vi "AllThingsBaxter_ROS.vi"() -> ()   [LabVIEW 2012]
uses:
  <userlib>/ROSforLV/ROS/MessageBuilding/std_msgs/subs/boolScalar.vi
  <userlib>/ROSforLV/ROS/MessageBuilding/std_msgs/subs/durationScalar.vi
  <userlib>/ROSforLV/ROS/MessageBuilding/std_msgs/subs/float32Scalar.vi
  <userlib>/ROSforLV/ROS/MessageBuilding/std_msgs/subs/float64Scalar.vi
  <userlib>/ROSforLV/ROS/MessageBuilding/std_msgs/subs/i8Scalar.vi
  <userlib>/ROSforLV/ROS/MessageBuilding/std_msgs/subs/i16Scalar.vi
  <userlib>/ROSforLV/ROS/MessageBuilding/std_msgs/subs/i32Scalar.vi
  <userlib>/ROSforLV/ROS/MessageBuilding/std_msgs/subs/i64Scalar.vi
  <userlib>/ROSforLV/ROS/MessageBuilding/std_msgs/subs/stringScalar.vi
  <userlib>/ROSforLV/ROS/MessageBuilding/std_msgs/subs/timeScalar.vi
  <userlib>/ROSforLV/ROS/MessageBuilding/std_msgs/subs/u8Scalar.vi
  <userlib>/ROSforLV/ROS/MessageBuilding/std_msgs/subs/u16Scalar.vi
  <userlib>/ROSforLV/ROS/MessageBuilding/std_msgs/subs/u32Scalar.vi
  <userlib>/ROSforLV/ROS/MessageBuilding/std_msgs/subs/u64Scalar.vi
  <userlib>/ROSforLV/ROS/Code/_ROSDefinition.vi
panel:
  out "ROS Master":string="192.168.1.110:11311"
  # "check for Baxter enabled over ROS"
  # "130.64.16.138"
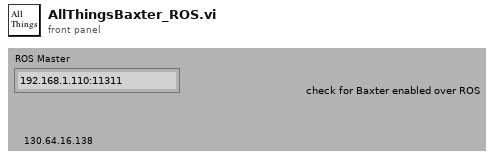
[diagram p1: front panel]
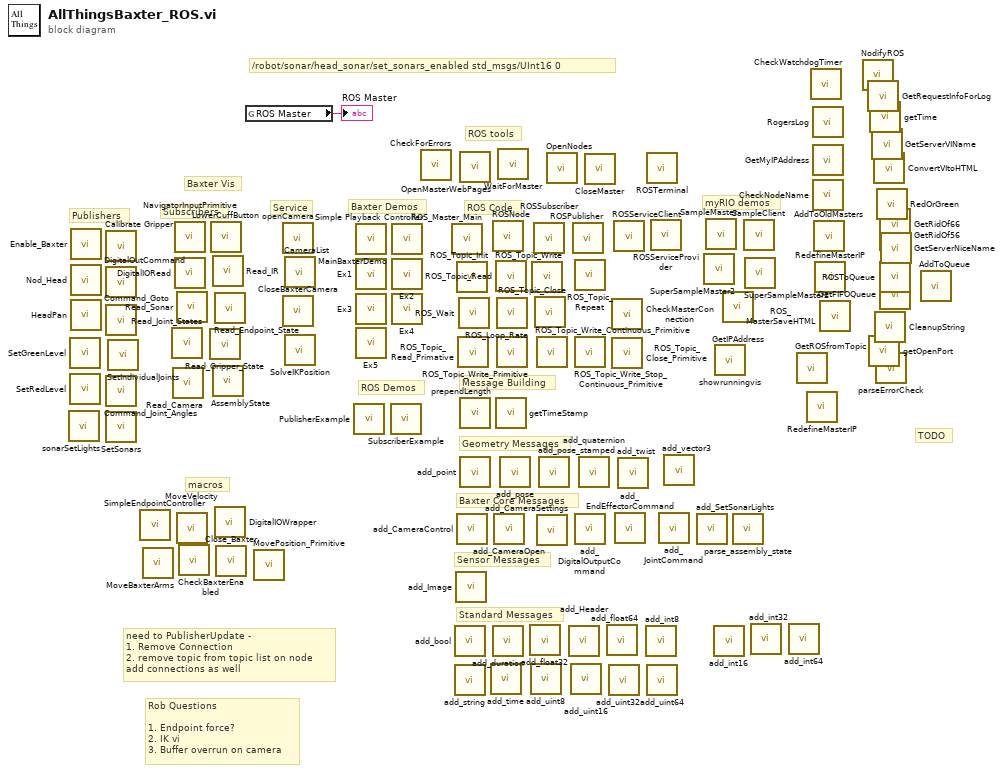
[diagram p0: block diagram]
diagram:
  # "myRIO demos"
  # "ROS Demos"
  # "/robot/sonar/head_sonar/set_sonars_enabled std_msgs/UInt16 0"
  # "ROS tools"
  # "TODO"
  # "macros"
  # "Service"
  # "Subscribers"
  # "Publishers"
  # "Standard Messages"
  # "Sensor Messages"
  # "Baxter Core Messages"
  # "Geometry Messages"
  # "Message Building"
  # "Rob Questions\n\n1. Endpoint force?\n2. IK vi\n3. Buffer overrun on camera"
  # "need to PublisherUpdate - \n1. Remove Connection\n2. remove topic from topic list on node\nadd connections as well"
  # "ROS Code"
  # "Baxter Demos"
  # "Baxter Vis"
  n1 = call <userlib>:"sonarSetLights.vi"() -> ()  [unwired: 4 in, 1 out]
  n2 = call <userlib>:"SetGreenLevel.vi"() -> ()  [unwired: 4 in, 1 out]
  n3 = call <userlib>:"SetRedLevel.vi"() -> ()  [unwired: 4 in, 1 out]
  n4 = call <userlib>:"Enable_Baxter.vi"() -> ()  [unwired: 4 in, 1 out]
  n5 = call <userlib>:"Nod_Head.vi"() -> ()  [unwired: 4 in, 1 out]
  n6 = call <userlib>:"HeadPan.vi"() -> ()  [unwired: 4 in, 1 out]
  n7 = call <userlib>:"Calibrate Gripper.vi"() -> ()  [unwired: 6 in, 1 out]
  n8 = call <userlib>:"DigitalOutCommand.vi"() -> ()  [unwired: 5 in, 1 out]
  n9 = call <userlib>:"Command_Goto.vi"() -> ()  [unwired: 6 in, 1 out]
  n10 = call <userlib>:"Command_Joint_Angles.vi"() -> ()  [unwired: 6 in, 1 out]
  n11 = call <userlib>:"SetSonars.vi"() -> ()  [unwired: 4 in, 1 out]
  n12 = call <userlib>:"SetIndividualJoints.vi"() -> ()  [unwired: 6 in, 1 out]
  n13 = call <userlib>:"SimpleEndpointController.vi"() -> ()  [unwired: 5 in, 1 out]
  n14 = call <userlib>:"MoveBaxterArms.vi"() -> ()  [unwired: 6 in, 1 out]
  n15 = call <userlib>:"Read_Joint_States.vi"() -> ()  [unwired: 3 in, 2 out]
  n16 = call <userlib>:"Read_Camera.vi"() -> ()  [unwired: 3 in, 2 out]
  n17 = call <userlib>:"NavigatorInputPrimitive.vi"() -> ()  [unwired: 3 in, 2 out]
  n18 = call <userlib>:"DigitalIORead.vi"() -> ()  [unwired: 3 in, 2 out]
  n19 = call <userlib>:"Read_Sonar.vi"() -> ()  [unwired: 3 in, 2 out]
  n20 = call <userlib>:"MoveVelocity.vi"() -> ()  [unwired: 6 in, 1 out]
  n21 = call <userlib>:"CheckBaxterEnabled.vi"() -> ()  [unwired: 4 in, 1 out]
  n22 = call <userlib>:"Read_Gripper_State.vi"() -> ()  [unwired: 3 in, 2 out]
  n23 = call <userlib>:"LowerCuffButton.vi"() -> ()  [unwired: 3 in, 2 out]
  n24 = call <userlib>:"Read_IR.vi"() -> ()  [unwired: 3 in, 2 out]
  n25 = call <userlib>:"AssemblyState.vi"() -> ()  [unwired: 3 in, 2 out]
  n26 = call <userlib>:"Read_Endpoint_State.vi"() -> ()  [unwired: 3 in, 2 out]
  n27 = call <userlib>:"DigitalIOWrapper.vi"() -> ()  [unwired: 3 in, 2 out]
  n28 = call <userlib>:"Close_Baxter.vi"() -> ()  [unwired: 4 in, 1 out]
  n29 = global read "_ROSDefinition.vi" "ROS Master"() -> (→"ROS Master":string)
  n30 = call <userlib>:"MovePosition_Primitive.vi"() -> ()  [unwired: 6 in, 1 out]
  n31 = call <userlib>:"openCamera.vi"() -> ()  [unwired: 4 in, 1 out]
  n32 = call <userlib>:"CloseBaxterCamera.vi"() -> ()  [unwired: 5 in, 1 out]
  n33 = call <userlib>:"CameraList.vi"() -> ()  [unwired: 2 in, 2 out]
  n34 = call <userlib>:"SolveIKPosition.vi"() -> ()  [unwired: 7 in, 1 out]
  n35 = call <userlib>:"PublisherExample.vi"() -> ()  [unwired: 12 in]
  n36 = call <userlib>:"MainBaxterDemo.vi"() -> ()  [unwired: 12 in]
  n37 = call <userlib>:"Ex1.vi"() -> ()  [unwired: 12 in]
  n38 = call <userlib>:"Ex3.vi"() -> ()  [unwired: 12 in]
  n39 = call <userlib>:"Ex5.vi"() -> ()  [unwired: 12 in]
  n40 = call <userlib>:"SubscriberExample.vi"() -> ()  [unwired: 12 in]
  n41 = call <userlib>:"Simple Playback Controller.vi"() -> ()  [unwired: 12 in]
  n42 = call <userlib>:"Ex2.vi"() -> ()  [unwired: 12 in]
  n43 = call <userlib>:"Ex4.vi"() -> ()  [unwired: 12 in]
  n44 = call <userlib>:"CheckForErrors.vi"() -> ()  [unwired: 2 in, 3 out]
  n45 = call <userlib>:"ROS_Master_Main.vi"() -> ()  [unwired: 4 in]
  n46 = call-poly <userlib>:"add_bool.vi"() -> ()  [unwired: 5 in, 1 out]
  n47 = call-poly <userlib>:"add_string.vi"() -> ()  [unwired: 5 in, 1 out]
  n48 = call <userlib>:"add_Image.vi"() -> ()  [unwired: 5 in, 1 out]
  n49 = call <userlib>:"ROS_Topic_Init.vi"() -> ()  [unwired: 2 in, 2 out]
  n50 = call <userlib>:"add_CameraControl.vi"() -> ()  [unwired: 5 in, 1 out]
  n51 = call <userlib>:"ROS_Topic_Read_Primative.vi"() -> ()  [unwired: 2 in, 3 out]
  n52 = call <userlib>:"ROS_Wait.vi"() -> ()  [unwired: 5 in, 2 out]
  n53 = call <userlib>:"OpenMasterWebPages.vi"() -> ()  [unwired: 4 in]
  n54 = call <userlib>:"prependLength.vi"() -> ()  [unwired: 5 in, 1 out]
  n55 = call <userlib>:"add_point.vi"() -> ()  [unwired: 5 in, 1 out]
  n56 = call-poly <userlib>:"add_time.vi"() -> ()  [unwired: 5 in, 1 out]
  n57 = call <userlib>:"ROSNode.vi"() -> ()  [unwired: 4 in]
  n58 = call-poly <userlib>:"add_duration.vi"() -> ()  [unwired: 5 in, 1 out]
  n59 = call <userlib>:"add_CameraOpen.vi"() -> ()  [unwired: 5 in, 1 out]
  n60 = call <userlib>:"ROS_Topic_Read.vi"() -> ()  [unwired: 3 in, 3 out]
  n61 = call <userlib>:"getTimeStamp.vi"() -> ()  [unwired: 2 in, 3 out]
  n62 = call <userlib>:"ROS_Loop_Rate.vi"() -> ()  [unwired: 5 in, 2 out]
  n63 = call <userlib>:"ROS_Topic_Write_Primitive.vi"() -> ()  [unwired: 3 in, 1 out]
  n64 = call <userlib>:"WaitForMaster.vi"() -> ()  [unwired: 1 in, 1 out]
  n65 = call <userlib>:"add_pose.vi"() -> ()  [unwired: 5 in, 1 out]
  n66 = call-poly <userlib>:"add_float32.vi"() -> ()  [unwired: 5 in, 1 out]
  n67 = call-poly <userlib>:"add_uint8.vi"() -> ()  [unwired: 5 in, 1 out]
  n68 = call <userlib>:"ROS_Topic_Write.vi"() -> ()  [unwired: 4 in, 2 out]
  n69 = call <userlib>:"ROSSubscriber.vi"() -> ()  [unwired: 4 in]
  n70 = call <userlib>:"ROS_Topic_Close.vi"() -> ()  [unwired: 4 in, 1 out]
  n71 = call <userlib>:"ROS_Topic_Write_Continuous_Primitive.vi"() -> ()  [unwired: 3 in, 1 out]
  n72 = call <userlib>:"add_CameraSettings.vi"() -> ()  [unwired: 5 in, 1 out]
  n73 = call <userlib>:"add_pose_stamped.vi"() -> ()  [unwired: 5 in, 1 out]
  n74 = call <userlib>:"OpenNodes.vi"() -> ()  [unwired: 2 in]
  n75 = call <userlib>:"add_Header.vi"() -> ()  [unwired: 5 in, 1 out]
  n76 = call-poly <userlib>:"add_uint16.vi"() -> ()  [unwired: 5 in, 1 out]
  n77 = call <userlib>:"ROSPublisher.vi"() -> ()  [unwired: 4 in]
  n78 = call <userlib>:"ROS_Topic_Repeat.vi"() -> ()  [unwired: 4 in, 2 out]
  n79 = call <userlib>:"ROS_Topic_Write_Stop_Continuous_Primitive.vi"() -> ()  [unwired: 3 in, 1 out]
  n80 = call <userlib>:"add_DigitalOutputCommand.vi"() -> ()  [unwired: 5 in, 1 out]
  n81 = call <userlib>:"add_quaternion.vi"() -> ()  [unwired: 5 in, 1 out]
  n82 = call <userlib>:"CloseMaster.vi"() -> ()  [unwired: 3 in, 1 out]
  n83 = call-poly <userlib>:"add_float64.vi"() -> ()  [unwired: 5 in, 1 out]
  n84 = call-poly <userlib>:"add_uint32.vi"() -> ()  [unwired: 5 in, 1 out]
  n85 = call <userlib>:"CheckMasterConnection.vi"() -> ()  [unwired: 2 in, 2 out]
  n86 = call <userlib>:"ROS_Topic_Close_Primitive.vi"() -> ()  [unwired: 3 in, 1 out]
  n87 = call <userlib>:"ROSServiceClient.vi"() -> ()  [unwired: 4 in]
  n88 = call <userlib>:"add_EndEffectorCommand.vi"() -> ()  [unwired: 5 in, 1 out]
  n89 = call <userlib>:"add_twist.vi"() -> ()  [unwired: 5 in, 1 out]
  n90 = call-poly <userlib>:"add_int8.vi"() -> ()  [unwired: 5 in, 1 out]
  n91 = call <userlib>:"ROSTerminal.vi"() -> ()  [unwired: 2 in]
  n92 = call-poly <userlib>:"add_uint64.vi"() -> ()  [unwired: 5 in, 1 out]
  n93 = call <userlib>:"ROSServiceProvider.vi"() -> ()  [unwired: 4 in]
  n94 = call <userlib>:"add_JointCommand.vi"() -> ()  [unwired: 11 in, 1 out]
  n95 = call <userlib>:"add_vector3.vi"() -> ()  [unwired: 5 in, 1 out]
  n96 = call <userlib>:"add_SetSonarLights.vi"() -> ()  [unwired: 5 in, 1 out]
  n97 = call <userlib>:"SuperSampleMaster2.vi"() -> ()  [unwired: 12 in]
  n98 = call <userlib>:"SampleMaster.vi"() -> ()  [unwired: 12 in]
  n99 = call-poly <userlib>:"add_int16.vi"() -> ()  [unwired: 5 in, 1 out]
  n100 = call <userlib>:"showrunningvis.vi"() -> ()  [unwired: 1 in]
  n101 = call <userlib>:"GetIPAddress.vi"() -> ()  [unwired: 3 in, 1 out]
  n102 = call <userlib>:"parse_assembly_state.vi"() -> ()  [unwired: 3 in, 3 out]
  n103 = call <userlib>:"SampleClient.vi"() -> ()  [unwired: 12 in]
  n104 = call <userlib>:"SuperSampleMaster2.vi"() -> ()  [unwired: 12 in]
  n105 = call-poly <userlib>:"add_int32.vi"() -> ()  [unwired: 5 in, 1 out]
  n106 = call-poly <userlib>:"add_int64.vi"() -> ()  [unwired: 5 in, 1 out]
  n107 = call <userlib>:"GetROSfromTopic.vi"() -> ()  [unwired: 3 in, 2 out]
  n108 = call <userlib>:"RedefineMasterIP.vi"() -> ()  [unwired: 2 in, 1 out]
  n109 = call <userlib>:"CheckWatchdogTimer.vi"() -> ()  [unwired: 6 in]
  n110 = call <userlib>:"RogersLog.vi"() -> ()  [unwired: 5 in, 2 out]
  n111 = call <userlib>:"GetMyIPAddress.vi"() -> ()  [unwired: 2 in, 2 out]
  n112 = call <userlib>:"CheckNodeName.vi"() -> ()  [unwired: 2 in, 2 out]
  n113 = call <userlib>:"AddToOldMasters.vi"() -> ()  [unwired: 4 in]
  n114 = call <userlib>:"RedefineMasterIP.vi"() -> ()  [unwired: 2 in, 1 out]
  n115 = call <userlib>:"ROS_MasterSaveHTML.vi"() -> ()  [unwired: 6 in]
  n116 = call <userlib>:"NodifyROS.vi"() -> ()  [unwired: 1 in, 1 out]
  n117 = call <userlib>:"GetRequestInfoForLog.vi"() -> ()  [unwired: 1 in, 1 out]
  n118 = call <userlib>:"getOpenPort.vi"() -> ()  [unwired: 1 out]
  n119 = call <userlib>:"getTime.vi"() -> ()  [unwired: 1 in, 1 out]
  n120 = call <userlib>:"GetServerVIName.vi"() -> ()  [unwired: 1 in, 1 out]
  n121 = call <userlib>:"ConvertVItoHTML.vi"() -> ()  [unwired: 1 in, 2 out]
  n122 = call <userlib>:"CleanupString.vi"() -> ()  [unwired: 1 in, 1 out]
  n123 = call <userlib>:"parseErrorCheck.vi"() -> ()  [unwired: 4 in, 1 out]
  n124 = call <userlib>:"RedOrGreen.vi"() -> ()  [unwired: 1 in, 1 out]
  n125 = call <userlib>:"GetRidOf66.vi"() -> ()  [unwired: 1 in, 1 out]
  n126 = call <userlib>:"GetRidOf56.vi"() -> ()  [unwired: 1 in, 1 out]
  n127 = call <userlib>:"ROSToQueue.vi"() -> ()  [unwired: 4 in, 2 out]
  n128 = call <userlib>:"GetFIFOQueue.vi"() -> ()  [unwired: 4 in, 2 out]
  n129 = call <userlib>:"GetServerNiceName.vi"() -> ()  [unwired: 2 in, 1 out]
  n130 = call <userlib>:"AddToQueue.vi"() -> ()  [unwired: 5 in, 1 out]
